vi "Int8Array Create.vi"(8 "error in (no error)":errorcluster, 11 "I8 array in":i8[](array[numeric])) -> (0 "error out":errorcluster, 3 "Int8Array DVR out":refnum<data-value>)   [LabVIEW 2015, in "MDSplus.lvlib"]
uses:
  <vilib>/MDSplus/Library/MDSplus.lvlib
  <vilib>/MDSplus/Classes/Data_Class/Array_Class/Int8Array_Class/Int8Array.lvclass
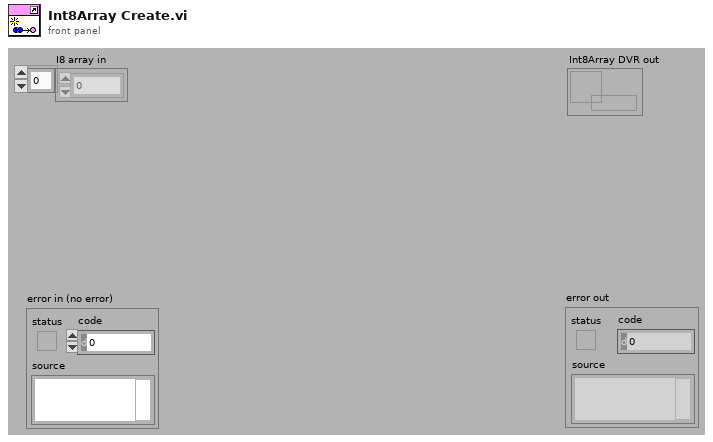
[diagram p1: front panel]
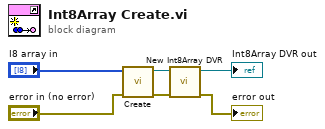
[diagram p0: block diagram]
diagram:
  n1 = call <vilib>:"Create.vi"("error in (no error)"="error in (no error)", "I8 array in"="I8 array in") -> ("error out"=w3:errorcluster, "Int8Array out"=w4:refnum<class "Int8Array.lvclass">)  [unwired: 8 in]
  n2 = call <vilib>:"New Int8Array DVR.vi"("error in (no error)"=w3, "Int8Array in"=w4) -> ("error out"=→"error out":errorcluster, "Int8Array DVR out"=→"Int8Array DVR out":refnum<data-value>)  [unwired: 8 in]
